vi "Initialize.vi"(4 "FIFO Options":T1, 5 "Status":refnum<class "Framework Status.lvclass">, 6 "id":i32, 7 "Logging Interface":refnum<class "Logging Interface.lvclass">, 8 "error in (no error)":errorcluster, 9 "Transfer Groups":refnum<class "Transfer Group.lvclass">[](array[class]), 10 "Components":refnum<class "Component.lvclass">[](array[class]), 11 "Plugin Configuration":refnum<class "Plugin Configuration.lvclass">) -> (0 "error out":errorcluster, 2 "Plugin Threads":refnum<class "Plugin Thread.lvclass">[](array[class]), 3 "Plugin out":refnum<class "Plugin.lvclass">)   [LabVIEW 2019, in "DSF Core.lvlib" / "Plugin.lvclass"]
uses:
  Plugin.lvclass
  Typedefs/DSF FIFO Options.ctl
  Component/Component.lvclass
  Configuration/Core/Plugin/Plugin Configuration.lvclass
  Thread/Plugin/Plugin Thread.lvclass
  C:/Dev/GitHub/niveristand-data-sharing-framework-custom-device/Core/Classes/Thread/Thread.lvclass
  Interface/Logging/Logging Interface.lvclass
  Framework Status/Framework Status.lvclass
  Transfer Group/Transfer Group.lvclass
  Framework Status/Framework Status.lvclass/Framework Status.ctl
  <vilib>/NI/Memory Manager/Classes/Pointer/Pointer.lvclass/Pointer.ctl
  Timing/Timing.lvclass/Timing.ctl
  Plugin.lvclass/Plugin.ctl
  Transfer Group/Transfer Group.lvclass/Transfer Group.ctl
  Transfer/Transfer.lvclass/Transfer.ctl
  Component/Component.lvclass/Component.ctl
  Interface/Interface.lvclass/Interface.ctl
  Thread/Thread.lvclass/Thread.ctl
  Thread/Plugin/Plugin Thread.lvclass/Plugin Thread.ctl
  Timing/Create Timing.vi
  Transfer Group/Set Inline.vi
  Transfer Group/Initialize Status.vi
  Transfer Group/Set ID.vi
  Configure Transfer Groups.vi
  Timing/Is Inline.vi
  Transceiver/New.vi
  Transfer Group/Subset Transfer Groups.vi
  Thread/Plugin/Find.vi
  Status/Subset Status.vi
  Framework Status/Get Plugin Subset.vi
  Timing/Set Decimation.vi
  Timing/Set Offset.vi
  Timing/Set Priority.vi
  Timing/Errors.vi
  Timing/Invalid Offset.vi
  Timing/Invalid Priority.vi
  Transfer/Set Inline.vi
  <vilib>/NI/Memory Manager/Classes/Pointer/Is Null.vi
  Status/Create.vi
  Transfer Group/Sort by Priority.vi
  Transfer Group/Separate Rx and Tx.vi
  Transfer Group/Separate Inline and Async.vi
  Thread/Set Thread Parameters.vi
  Thread/Set Name.vi
  Get Timing.vi
  Timing/Get Priority.vi
  Get ID.vi
  Get Name.vi
  Thread/Set ID.vi
  Interface/Plugin/Create.vi
  Transfer Group/Get ID.vi
  <vilib>/Utility/error.llb/Clear Errors.vi
  Component/Get Objects.vi
  <vilib>/NI/Memory Manager/Classes/Pointer/Subset.vi
  Status/Status Size.vi
  Timing/New Timing Error.vi
  <vilib>/NI/Memory Manager/VIs/Write String to Source.vi
  <vilib>/NI/Memory Manager/VIs/Write Numeric to Source.vi
  <vilib>/NI/Memory Manager/VIs/Write Numeric Scalar to Source (Base10 U64).vi
  Timing/Get Decimation.vi
  <vilib>/NI/Memory Manager/Classes/Pointer/Get Address.vi
  <vilib>/NI/Memory Manager/Classes/Pointer/Allocate.vi
  Status/Write Status 1D.vi
  Transfer Group/Get Direction.vi
  Transfer Group/Get Timing.vi
  Transfer Group/Set Active.vi
  Interface/New Interface.vi
  <vilib>/NI/Memory Manager/Classes/Pointer/Encapsulate.vi
  <vilib>/NI/Memory Manager/Classes/Pointer/Check Null Pointer.vi
  <vilib>/NI/Memory Manager/Classes/Pointer/Check Length.vi
  <vilib>/NI/Memory Manager/VIs/New Error Cluster.vi
  <vilib>/NI/Memory Manager/VIs/New Error Cluster (512B).vi
  <vilib>/NI/Memory Manager/VIs/Set Error Code.vi
  <vilib>/NI/Memory Manager/VIs/Set Error Status.vi
  <vilib>/NI/Memory Manager/VIs/Set Error Source.vi
  VIs/Constants/Constants.vi
  VIs/Constants/Engine Library Name.vi
  Timing/Timing Error Info.vi
  <vilib>/NI/Memory Manager/Classes/Pointer/Set Address.vi
  <vilib>/NI/Memory Manager/Classes/Pointer/Set Size.vi
  <vilib>/NI/Memory Manager/Classes/Pointer/Set Internal.vi
  <vilib>/NI/Memory Manager/Classes/Pointer/Check Size.vi
  Interface/Create RT FIFO.vi
  <vilib>/NI/Memory Manager/Classes/Pointer/Errors.vi
  <vilib>/NI/Memory Manager/Classes/Pointer/Null Pointer.vi
  <vilib>/NI/Memory Manager/Classes/Pointer/Get Size.vi
  <vilib>/NI/Memory Manager/Classes/Pointer/Check Bounds (Pointer).vi
  VIs/Constants/Base Error Code.vi
  Timing/Base Error Offset.vi
  <vilib>/NI/Memory Manager/Classes/Pointer/Out of Bounds.vi
  <vilib>/NI/Memory Manager/Classes/Pointer/Create Error.vi
  <vilib>/NI/Memory Manager/Classes/Pointer/Write Pointer Size to Error.vi
  <vilib>/NI/Memory Manager/Constants/Constants.vi
  <vilib>/NI/Memory Manager/Constants/Library Name.vi
  <vilib>/NI/Memory Manager/Classes/Pointer/Pointer Error Info.vi
  <vilib>/NI/Memory Manager/Constants/Pointer Class Name.vi
  Status/Status Pointer.lvclass
  C:/Program Files (x86)/National Instruments/LabVIEW 2019/vi.lib/NI/Memory Manager/Classes/Pointer/Pointer.lvclass
  Thread/Plugin/Transceiver/Transceiver Thread.lvclass
  C:/Dev/GitHub/niveristand-data-sharing-framework-custom-device/Core/Classes/Thread/Plugin/Plugin Thread.lvclass
  Interface/Plugin/Plugin Interface.lvclass
  C:/Dev/GitHub/niveristand-data-sharing-framework-custom-device/Core/Classes/Interface/Interface.lvclass
  Configuration/Core/Plugin/Get Thread Configurations.vi
  Configuration/Core/Thread/Get Core Configuration.vi
  Timing/Timing.lvclass
  Configuration/Core/Thread/Thread Configuration.lvclass
  Framework/Framework.lvclass
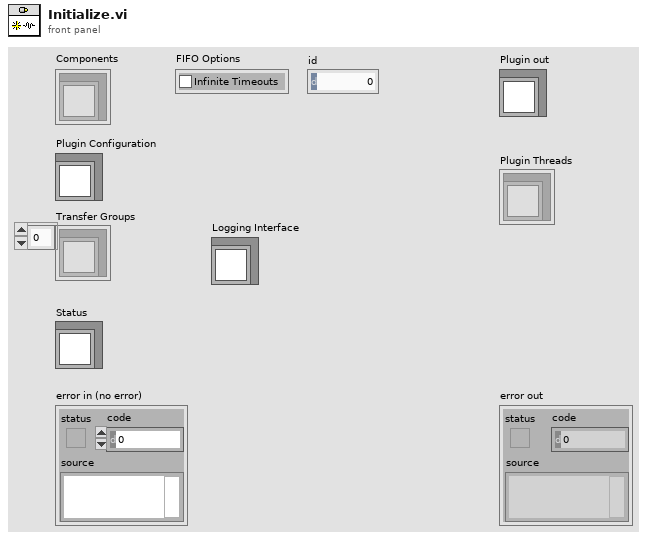
[diagram p1: front panel]
types:
  T1 = typedef "DSF Core.lvlib/Framework.lvclass/DSF FIFO Options.ctl" = cluster{"Infinite Timeouts":bool}
  T2 = typedef "DSF Core.lvlib/Plugin Configuration.lvclass/Core Plugin Configuration.ctl" = cluster{"name":string, "components":string[], "cycle timing":T3}
  T3 = typedef "DSF Core.lvlib/DSF Timing Info.ctl" = cluster{"priority":u64, "decimation":u64, "offset":u64}
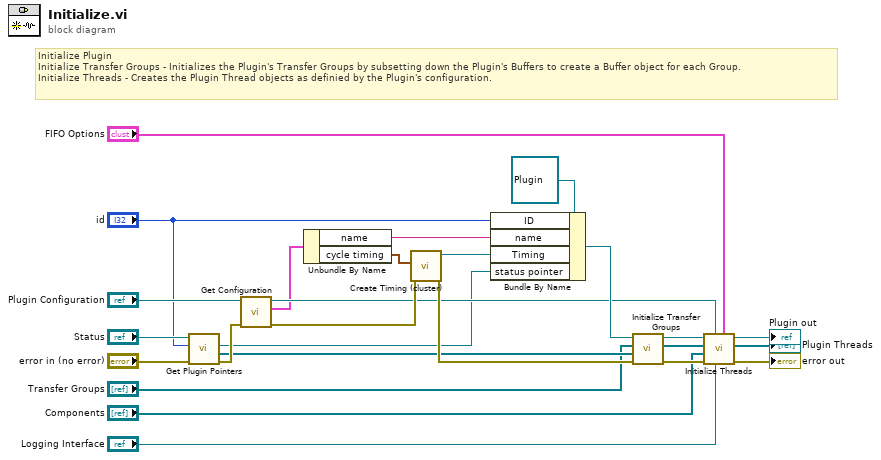
[diagram p0: block diagram]
diagram:
  # "Initialize Plugin\nInitialize Transfer Groups - Initializes the Plugin's Transfer Groups by subsetting down the Plugin's Buffers to create a Buffer object for each Group.\nInitialize Threads - Creates the Plugin Thread objects as definied by the Plugin's configuration."
  n1 = call "Get Plugin Pointers.vi"("error in (no error)"="error in (no error)", "plugin index"="id", "Framework Status in"="Status") -> ("error out"=w8:errorcluster, "group status pointers"=w4:refnum<class "Status Pointer.lvclass">[], "plugin status pointer"=w5:refnum<class "Status Pointer.lvclass">)  [unwired: 5 in, 1 out]
  n2 = call "Get Configuration.vi"("error in (no error)"=w8, "Core Plugins Configuration in"="Plugin Configuration") -> ("error out"=w7:errorcluster, "configuration"=w2:T2, "Core Plugins Configuration out"=w6:refnum<class "Plugin Configuration.lvclass">)  [unwired: 7 in]
  n3 = Unbundle By Name(w2) -> ("name"=w14:string, "cycle timing"=w13:T3)
  n4 = call "Create Timing (cluster).vi"("error in (no error)"=w7, "cycle timing"=w13) -> ("error out"=w17:errorcluster, "Timing"=w20:refnum<class "Timing.lvclass">)  [unwired: 8 in]
  n5 = Bundle By Name(cluster=refnum<class "Plugin.lvclass"> refnum ("DSF Core.lvlib:Plugin"), "ID"="id", "name"=w14, "Timing"=w20, "status pointer"=w5) -> (w19:refnum<class "Plugin.lvclass">)
  n6 = call "Initialize Transfer Groups.vi"("error in (no error)"=w17, "group status pointers"=w4, "Transfer Groups in"="Transfer Groups", "Plugin in"=w19) -> ("error out"=w23:errorcluster, "Transfer Groups out"=w15:refnum<class "Transfer Group.lvclass">[], "Plugin out"=w25:refnum<class "Plugin.lvclass">)  [unwired: 5 in]
  n7 = call "Initialize Threads.vi"("FIFO Options"="FIFO Options", "Logging Interface"="Logging Interface", "Plugin Configuration"=w6, "error in (no error)"=w23, "Components"="Components", "Transfer Groups"=w15, "Plugin in"=w25) -> ("error out"=→"error out":errorcluster, "Plugin Threads"=→"Plugin Threads":refnum<class "Plugin Thread.lvclass">[], "Plugin out"=→"Plugin out":refnum<class "Plugin.lvclass">)  [unwired: 2 in]
